vi "dfd_Alternate Sign of Polynomial.vi"(0 "polynomial in":dbl[](array[numeric]), 1 "even? (F)":bool) -> (2 "polynomial out":dbl[](array[numeric]))   [LabVIEW 2017, in "NI_DigFilterLicensed.lvlib"]
uses:
  <vilib>/addons/Digital Filter Design/NI_DigFilterLicensed.lvlib
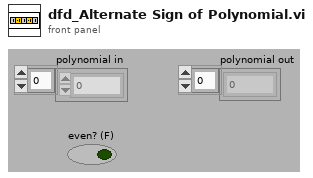
[diagram p1: front panel]
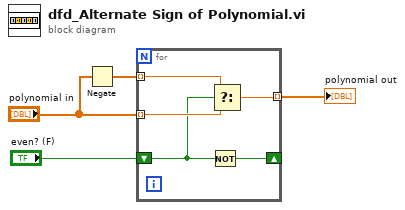
[diagram p0: block diagram]
diagram:
  n1 = Negate(x="polynomial in") -> (-x=w3:dbl[])
  n2 = for {
    shift-right: [w5] -> _
    shift-left: "even? (F)" -> [w6]
    tunnel: "polynomial in" -> [w8] mode=indexing
    tunnel: w3 -> [w9] mode=indexing
    tunnel: [w7] -> w1 mode=indexing
    n3 = Not(x=w6) -> (.not. x?=w5:bool)
    n4 = Select(t=w9, s=w6, f=w8) -> (s? t:f=w7:dbl)
  }
  "polynomial out" <- w1
